vi "InitTank.vi"(8 "Error In":errorcluster) -> (0 "Error Out":errorcluster, 3 "BactaTank out":refnum<class "BactaTank.lvclass">)   [LabVIEW 2021, in "BactaTank.lvclass"]
uses:
  BactaTank.lvclass
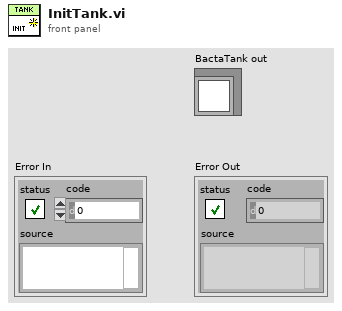
[diagram p1: front panel]
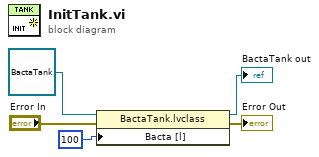
[diagram p0: block diagram]
diagram:
  n1 = property class="BactaTank.lvclass"(reference=refnum<class "BactaTank.lvclass"> refnum, error in="Error In", "Bacta [l]"=u8 100) -> (reference out=→"BactaTank out":refnum<class "BactaTank.lvclass">, error out=→"Error Out":errorcluster)
